vi "Start Sync.vi"(8 "error in (no error)":errorcluster, 11 "gRPC service in":refnum<class "ExamplePluginOOBService.lvclass">) -> (0 "error out":errorcluster, 3 "gRPC service out":refnum<class "ExamplePluginOOBService.lvclass">)   [LabVIEW 2025, in "ExamplePluginOOBService_server.lvlib" / "ExamplePluginOOBService.lvclass"]
uses:
  ExamplePluginOOBService.lvclass
  ExamplePluginOOBService.lvclass/ExamplePluginOOBService.ctl
  Example Plugin.lvclass
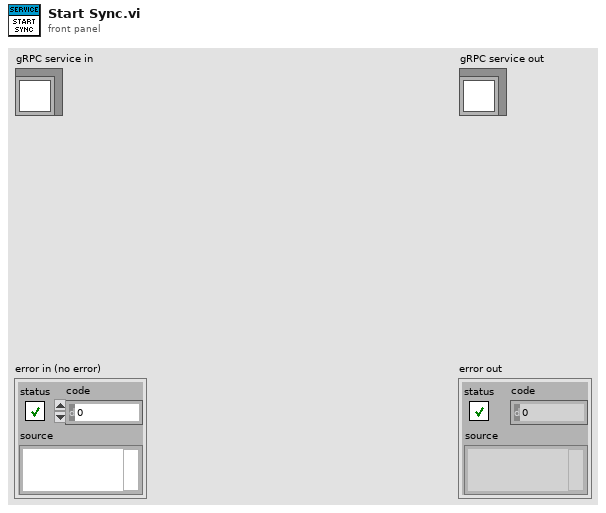
[diagram p1: front panel]
types:
  T1 = typedef "ExamplePluginOOBService_server.lvlib/ExamplePluginOOBService.lvclass/Server Internal UEs.ctl" = cluster{"ExamplePluginOOBService PauseResume Internal UE":refnum<user-event>, "ExamplePluginOOBService Export Internal UE":refnum<user-event>}
  T2 = typedef "ExamplePluginOOBService_server.lvlib/ExamplePluginOOBService.lvclass/Server gRPC UEs.ctl" = cluster{"ExamplePluginOOBService PauseResume gRPC UE":refnum<user-event>, "ExamplePluginOOBService Export gRPC UE":refnum<user-event>}
  T3 = typedef "grpc-lvsupport-release.lvlib/grpcId.ctl" = u64
  T4 = typedef "ExamplePluginOOBService_server.lvlib/hwval_BoolRequest.ctl" = cluster{"BooleanData":bool}
  T5 = typedef "Example Plugin.lvclass/OOB to Logic Data.ctl" = cluster{"PauseResume":bool, "Export":string}
  T6 = typedef "ExamplePluginOOBService_server.lvlib/hwval_ExportRequest.ctl" = cluster{"FileType":string}
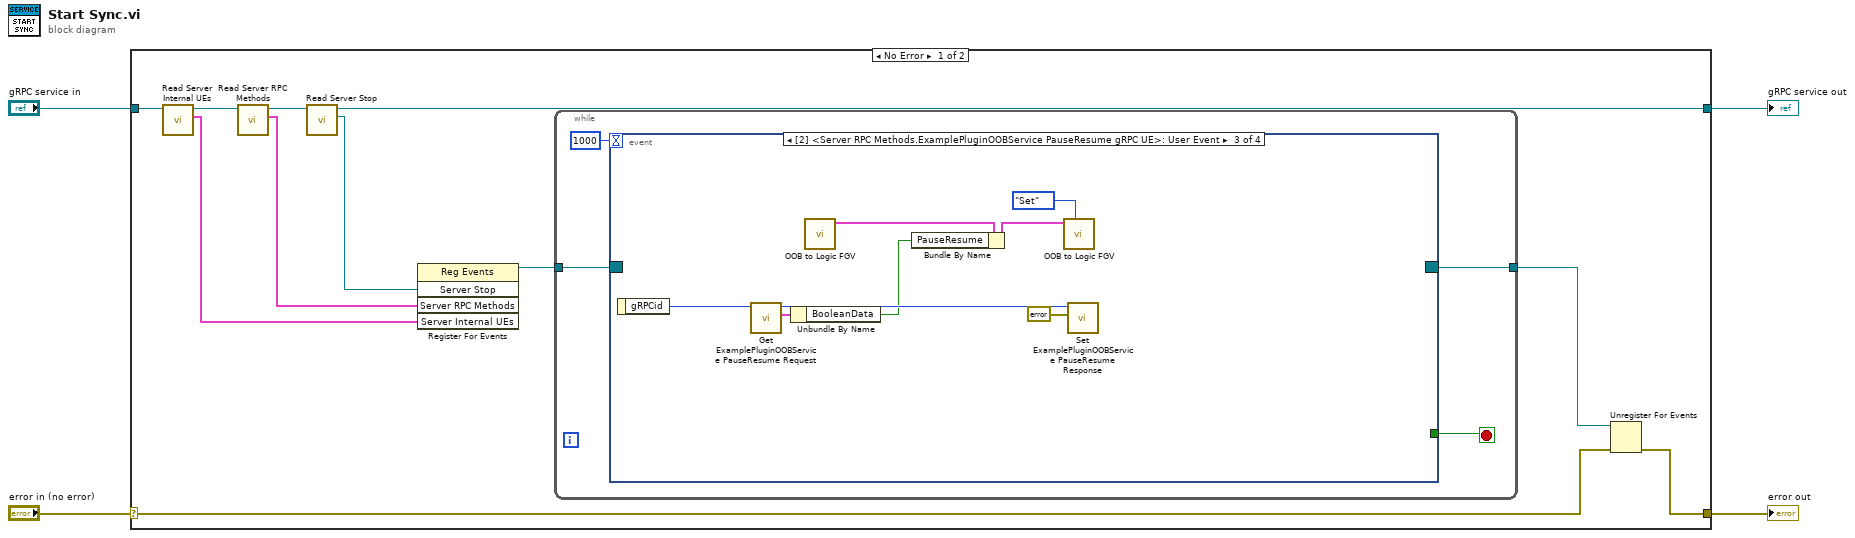
[diagram p0: block diagram]
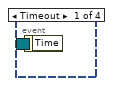
[diagram p2: hidden frame]
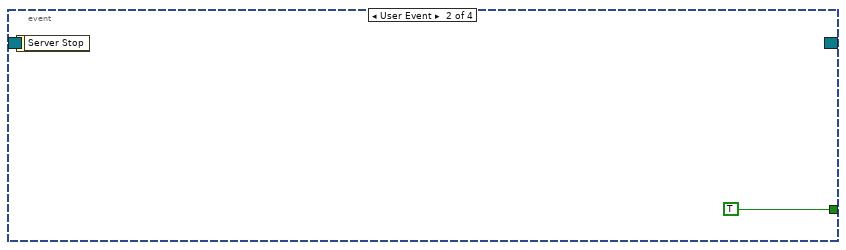
[diagram p3: hidden frame]
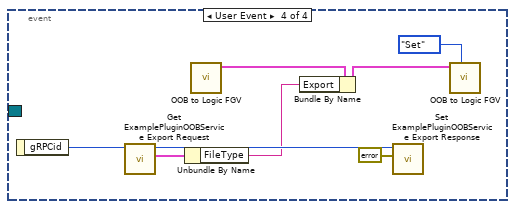
[diagram p4: hidden frame]
diagram:
  n1 = case shown="No Error" "error in (no error)" {
    selector: "error in (no error)" -> [w9 w38]
    tunnel: [w8 w38] -> w3
    tunnel: [w6 w37] -> w1
    tunnel: "gRPC service in" -> [w15 w37]
    frame No Error {
      n2 = call "Read Server Internal UEs.vi"("gRPC service in"=w15) -> ("Server Internal UEs"=w13:T1, "gRPC service out"=w14:refnum<class "ExamplePluginOOBService.lvclass">)  [unwired: 8 in, 1 out]
      n3 = call "Read Server RPC Methods.vi"("gRPC service in"=w14) -> ("Server RPC Methods"=w7:T2, "gRPC service out"=w12:refnum<class "ExamplePluginOOBService.lvclass">)  [unwired: 8 in, 1 out]
      n4 = call-dynamic "Read Server Stop.vi"("gRPC service in"=w12) -> ("Server Stop"=w5:refnum<user-event>, "gRPC service out"=w6:refnum<class "ExamplePluginOOBService.lvclass">)  [unwired: 8 in, 1 out]
      n5 = register-events(w5, w7, w13) -> (reference out=w11:refnum<event-registration>)  [unwired: 2 in, 1 out]
      n6 = while {
        tunnel: w11 -> [w16]
        tunnel: [w18] -> w10
        stop <- w19 stop-if-true
        n7 = event "RPC Methods Event Structure" shown="[2] <Server RPC Methods.ExamplePluginOOBService PauseResume gRPC UE>: User Event" {
          selector: w16 -> [_ _ _ _]
          dyn-events: [_ _ _ _] -> w18
          timeout: 1000 -> [_ _ _ _]
          tunnel: [_ TRUE _ _] -> w19
          event Timeout {
            n8 = event-data() -> ()  [unwired: 1 in, 1 out]
          }
          event User Event {
            n9 = event-data() -> ()  [unwired: 1 in, 1 out]
          }
          event User Event {
            n10 = event-data() -> ("gRPCid"=w25:T3)  [unwired: 1 in]
            n11 = call "Get ExamplePluginOOBService PauseResume Request.vi"("gRPCid"=w25) -> ("Message Data"=w22:T4, "gRPCid out"=w23:T3)  [unwired: 8 in, 1 out]
            n12 = Unbundle By Name(w22) -> ("BooleanData"=w21:bool)
            n13 = call "OOB to Logic FGV.vi"() -> ("OOB to Logic Data out"=w27:T5)  [unwired: 10 in, 1 out]
            n14 = Bundle By Name(cluster=w27, "PauseResume"=w21) -> (w26:T5)
            n15 = call "OOB to Logic FGV.vi"("Op (Get)"=enum16{"Get", "Set"}."Set", "OOB to Logic Data in"=w26) -> ()  [unwired: 8 in, 2 out]
            n16 = call "Set ExamplePluginOOBService PauseResume Response.vi"("Message Data"=errorcluster {"status"=FALSE, "code"=0, "source"=""} ("error in (no error)"), "gRPCid in"=w23) -> ()  [unwired: 9 in, 1 out]
          }
          event User Event {
            n17 = event-data() -> ("gRPCid"=w36:T3)  [unwired: 1 in]
            n18 = call "Get ExamplePluginOOBService Export Request.vi"("gRPCid"=w36) -> ("Message Data"=w30:T6, "gRPCid out"=w35:T3)  [unwired: 8 in, 1 out]
            n19 = Unbundle By Name(w30) -> ("FileType"=w29:string)
            n20 = call "OOB to Logic FGV.vi"() -> ("OOB to Logic Data out"=w32:T5)  [unwired: 10 in, 1 out]
            n21 = Bundle By Name(cluster=w32, "Export"=w29) -> (w31:T5)
            n22 = call "Set ExamplePluginOOBService Export Response.vi"("Message Data"=errorcluster {"status"=FALSE, "code"=0, "source"=""} ("error in (no error)"), "gRPCid in"=w35) -> ()  [unwired: 9 in, 1 out]
            n23 = call "OOB to Logic FGV.vi"("Op (Get)"=enum16{"Get", "Set"}."Set", "OOB to Logic Data in"=w31) -> ()  [unwired: 8 in, 2 out]
          }
        }
      }
      n24 = Unregister For Events(event registration refnum=w10, error in=w9) -> (error out=w8:errorcluster)
    }
    frame Error {
    }
  }
  "error out" <- w3
  "gRPC service out" <- w1
